vi "sub_log-header-write.vi"(7 "cmd":T1, 8 "error in (no error)":errorcluster, 11 "시험명":string) -> (0 "error out":errorcluster)   [LabVIEW 2019]
uses:
  log save type.ctl
  SubVIs/common/cmd_tablecnt.ctl
  _ctrl/rw.ctl
  _ctrl/create-rw-close.ctl
  Data Process/type-data.ctl
panel:
  out "Array":path[](array[path])
  out "dup path":path
  out "appended path":path
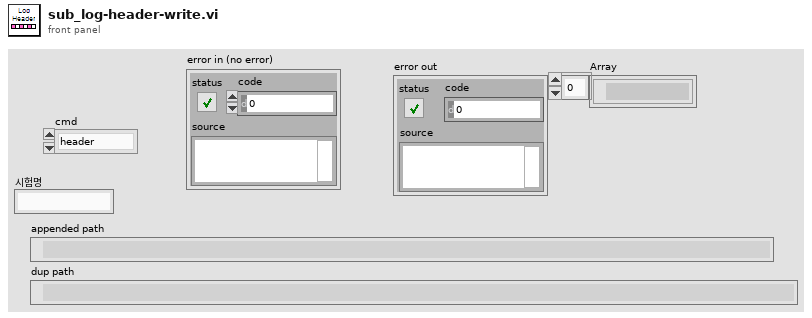
[diagram p1: front panel]
types:
  T1 = typedef "log save type.ctl" = enum16{"header", "data"}
  T2 = typedef "rw.ctl" = enum16{"read", "write"}
  T3 = typedef "cmd_tablecnt.ctl" = enum16{"Create", "Inital", "Write", "Default"}
  T4 = typedef "cap_config.ctl" = cluster{"Test Mode":enum32{"6.3.2 저온 작동/방치 시험", "6.3.3 고온 작동/방치 시험", "6.3.4 온도 싸이클 시험", "6.3.6 온습도 싸이클 시험", "6.3.8 결로 시험", "6.3.9 빙결 시험"}, "ON time[ms]":dbl, "OFF time[ms]":dbl, "1. 작동시간[분]":dbl, "2. 미작동시간[분]":dbl, "3. 작동시간[분]":dbl, "level[V]":dbl, "duty":dbl, "Freq":dbl, "Voltage+[V]":dbl, "Voltage-[V]":dbl, "Current+[A]":dbl, "Current-[A]":dbl, "출력전압[V]":dbl, "출력전류[A]":dbl, "OVP Level":dbl, "OCP Level":dbl, "Time Div":u16, "Record Len":i32, "방전 기준[V]":dbl, "Repeate (Each Ch)":u32, "Cycle[N]":u32, "ON/OFF 회 수[N]":dbl, "TrigPos[%]":dbl, "시험시간[분]":dbl}
  T5 = enum32{"6.3.2 저온 작동/방치 시험", "6.3.3 고온 작동/방치 시험", "6.3.4 온도 싸이클 시험", "6.3.6 온습도 싸이클 시험", "6.3.8 결로 시험", "6.3.9 빙결 시험"}
  T6 = typedef "Testing-info.ctl" = cluster{"전체채널수":u8, "현재채널번호":u8, "Irms":dbl, "입력전압":dbl, "입력전류":dbl, "출력전압":dbl, "출력전류":dbl, "온도":dbl, "제어단 단선":bool, "제어단 단락":bool, "제어단 특성변화":bool, "출력단 단선":bool, "출력단 단락":bool, "출력단 특성변화":bool, "출력단 전압":bool, "카운트 일치":bool, "Irms 판정":bool, "온도":bool, "테스트 회수":u32, "TestType":T7, "현재회수":u32, "Ch selection":cluster{"1ch":bool, "2ch":bool, "3ch":bool, "4ch":bool, "5ch":bool, "6ch":bool}, "반복":u32, "Path":path, "파일생성주기":u32, "start time":dbl, "stop time":dbl, "현재반복회수":u32, "NG":cluster{"입출력 카운트":bool, "출력전류RMS":bool}}
  T7 = typedef "sequence_single.ctl" = enum16{"Register", "RC", "B1", "B2", "B3", "Oper_LV", "Oper_HV", "ContR_LV"}
  T8 = typedef "type-data.ctl" = cluster{"dup path":path, "data":string}
  T9 = typedef "create-rw-close.ctl" = enum16{"create", "write", "read", "delete", "close"}
  T10 = cluster{"1ch":bool, "2ch":bool, "3ch":bool, "4ch":bool, "5ch":bool, "6ch":bool}
  T11 = typedef "result-path.ctl" = cluster{"Path-arr":path[]}
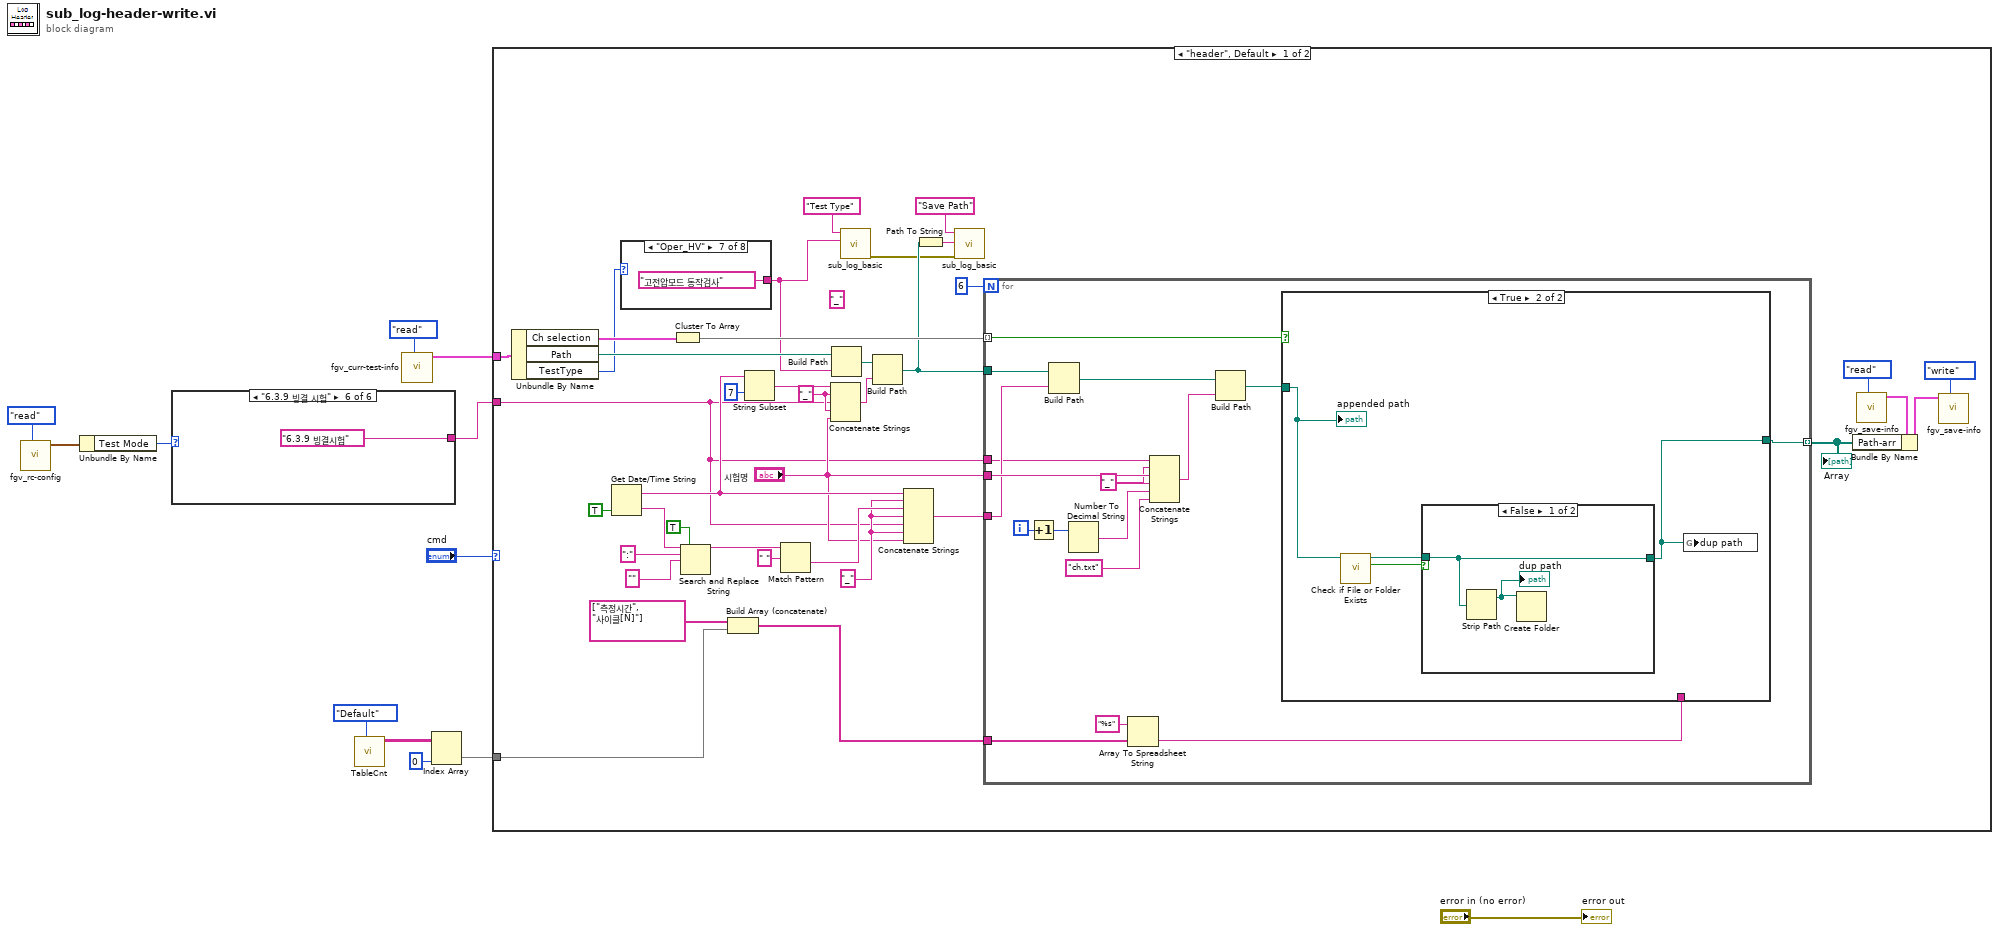
[diagram p0: block diagram]
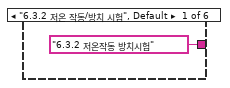
[diagram p2: hidden frame]
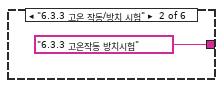
[diagram p3: hidden frame]
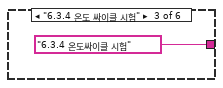
[diagram p4: hidden frame]
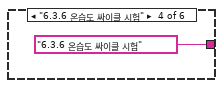
[diagram p5: hidden frame]
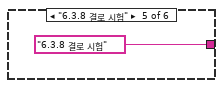
[diagram p6: hidden frame]
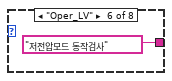
[diagram p12: hidden frame]
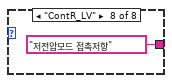
[diagram p13: hidden frame]
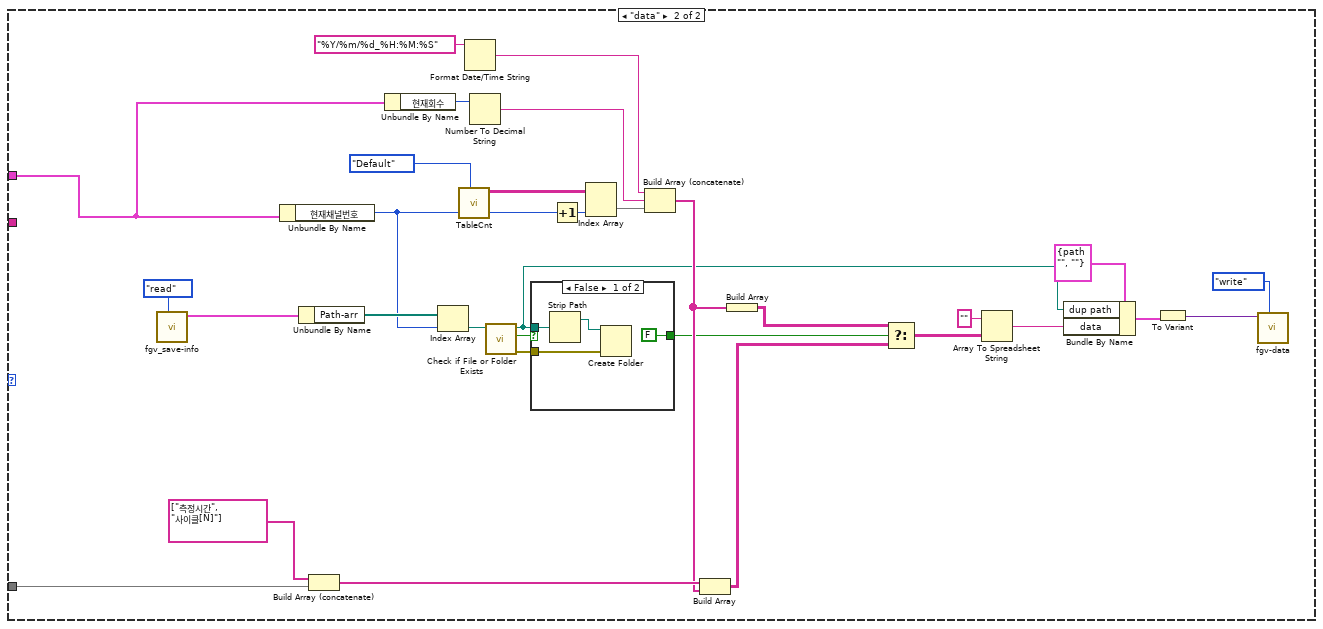
[diagram p16: hidden frame]
diagram:
  n1 = call "fgv_rc-config.vi"("cmd"=rw."read") -> ("Testconfig out"=w4:T4)  [unwired: 9 in, 1 out]
  n2 = Unbundle By Name(w4) -> ("Test Mode"=w2:T5)
  n3 = case shown="\"6.3.9 빙결 시험\"" w2 {
    tunnel: ["6.3.2 저온작동 방치시험" "6.3.3 고온작동 방치시험" "6.3.4 온도싸이클 시험" "6.3.6 온습도 싸이클 시험" "6.3.8 결로 시험" "6.3.9 빙결시험"] -> w1
    frame "6.3.2 저온 작동/방치 시험", Default {
    }
    frame "6.3.3 고온 작동/방치 시험" {
    }
    frame "6.3.4 온도 싸이클 시험" {
    }
    frame "6.3.6 온습도 싸이클 시험" {
    }
    frame "6.3.8 결로 시험" {
    }
    frame "6.3.9 빙결 시험" {
    }
  }
  n4 = call "TableCnt.vi"("cnt"=cmd_tablecnt."Default") -> ("Item Names"=w11:string[][])  [unwired: 9 in, 1 out]
  n5 = call "fgv_curr-test-info.vi"("cmd"=rw."read") -> ("현재테스트 정보 2"=w5:T6)  [unwired: 10 in]
  n6 = Index Array(array=w11, index (col)=0 ("disabled index (col)")) -> (element=w8:string[])  [unwired: 1 in]
  n7 = case shown="\"header\", Default" "cmd" {
    tunnel: w8 -> [w49 w104]
    tunnel: w5 -> [w27 w85]
    tunnel: w1 -> [w19 _]
    frame "header", Default {
      (unwired) "_" ("string")
      w24 = "_" ("string")
      w21 = "_" ("string")
      n8 = Unbundle By Name(w27) -> ("Ch selection"=w47:T10, "Path"=w38:path, "TestType"=w26:T7)
      n9 = Get Date/Time String(want seconds? (F)=TRUE) -> (date string=w23:string, time string=w45:string)  [unwired: 2 in]
      n10 = case shown="\"Oper_HV\"" w26 {
        tunnel: [_ _ _ _ _ "저전압모드 동작검사" ("Title") "고전압모드 동작검사" ("Title") "저전압모드 접촉저항" ("Title")] -> w25
        frame "Register", Default {
        }
        frame "RC" {
        }
        frame "B1" {
        }
        frame "B2" {
        }
        frame "B3" {
        }
        frame "Oper_LV" {
        }
        frame "Oper_HV" {
        }
        frame "ContR_LV" {
        }
      }
      n11 = Cluster To Array(cluster=w47) -> (array=w48:bool[])
      n12 = Search and Replace String(replace all?=TRUE ("replace all? (F)"), input string=w45, search string=":", replace string="" ("replace string (\"\")")) -> (result string=w41:string)  [unwired: 4 in, 3 out]
      n13 = Build Array (concatenate)(string[] ["측정시간", "사이클[N]"], w49) -> (w50:string[])
      n14 = String Subset(string=w23, length (rest)=7 ("length (rest)")) -> (substring=w30:string)  [unwired: 1 in]
      n15 = Match Pattern(string=w41, regular expression=" ") -> (after substring=w22:string)  [unwired: 1 in, 3 out]
      n16 = Concatenate Strings(w30, w24, w19, w24, "시험명") -> (w29:string)
      n17 = Build Path(base path=w38, name or relative path=w25) -> (appended path=w37:path)
      n18 = call "sub_log_basic.vi"("desc"=w25, "Title"="Test Type") -> ("error out"=w32:errorcluster)  [unwired: 9 in]
      n19 = Build Path(base path=w37, name or relative path=w29) -> (appended path=w34:path)
      n20 = Concatenate Strings(w23, w21, w22, w21, w19, w21, "시험명") -> (w28:string)
      n21 = Path To String(path=w34) -> (string=w35:string)
      n22 = call "sub_log_basic.vi"("error in"=w32, "desc"=w35, "Title"="Save Path") -> ()  [unwired: 8 in, 1 out]
      n23 = for {
        N: 6 -> [_]
        tunnel: w34 -> [w65]
        tunnel: [w67] -> w55 mode=indexing
        tunnel: w50 -> [w71]
        tunnel: w48 -> [w68] mode=indexing
        tunnel: "시험명" -> [w63]
        tunnel: w28 -> [w62]
        tunnel: w19 -> [w61]
        i -> [w76]
        w60 = "_" ("string")
        n24 = Increment(x=w76) -> (x+1=w69:i32)
        n25 = Build Path(base path=w65, name or relative path=w62) -> (appended path=w66:path)
        n26 = Number To Decimal String(number=w69) -> (decimal integer string=w75:string)  [unwired: 1 in]
        n27 = Array To Spreadsheet String(array=w71, 3:"%s" ("format string")) -> (spreadsheet string=w72:string)  [unwired: 1 in]
        n28 = Concatenate Strings(w61, w60, w63, w60, w75, "ch.txt" ("string")) -> (w64:string)
        n29 = Build Path(base path=w66, name or relative path=w64) -> (appended path=w73:path)
        n30 = case shown="True" w68 {
          tunnel: w73 -> [w77 w79]
          tunnel: w72 -> [_ _]
          tunnel: [w77 w78] -> w67
          frame False {
          }
          frame True {
            n31 = call <vilib>:"Check if File or Folder Exists.vi"("path"=w79) -> ("file or folder exists?"=w81:bool, "dup path"=w80:path)  [unwired: 8 in, 1 out]
            n32 = case shown="False" w81 {
              tunnel: w80 -> [w82 w84]
              tunnel: [w82 w84] -> w78
              frame False {
                n33 = Strip Path(path=w82) -> (stripped path=w83:path)  [unwired: 1 out]
                "dup path" <- w83
                n34 = Create Folder(path (use dialog)=w83) -> ()  [unwired: 2 in, 3 out]
              }
              frame True {
              }
            }
            n35 = global write "Global_내구.vi" "dup path"(w78) -> ()
            "appended path" <- w79
          }
        }
      }
      "Array" <- w55
      n36 = call "fgv_save-info.vi"("cmd"=rw."read") -> ("save info 2"=w54:T11)  [unwired: 10 in]
      n37 = Bundle By Name(cluster=w54, "Path-arr"=w55) -> (w56:T11)
      n38 = call "fgv_save-info.vi"("cmd"=rw."write", "save info"=w56) -> ()  [unwired: 9 in, 1 out]
    }
    frame "data" {
      n39 = call "fgv_save-info.vi"("cmd"=rw."read") -> ("save info 2"=w114:T11)  [unwired: 10 in]
      n40 = Unbundle By Name(w85) -> ("현재채널번호"=w109:u8)
      n41 = Unbundle By Name(w114) -> ("Path-arr"=w113:path[])
      n42 = Build Array (concatenate)(string[] ["측정시간", "사이클[N]"], w104) -> (w103:string[])
      n43 = Unbundle By Name(w85) -> ("현재회수"=w107:u32)
      n44 = Index Array(array=w113, index=w109) -> (element=w105:path)
      n45 = call "TableCnt.vi"("cnt"=cmd_tablecnt."Default") -> ("Item Names"=w110:string[][])  [unwired: 9 in, 1 out]
      n46 = Format Date/Time String(time format string (%c)="%Y/%m/%d_%H:%M:%S") -> (date/time string=w86:string)  [unwired: 2 in]
      n47 = Number To Decimal String(number=w107) -> (decimal integer string=w87:string)  [unwired: 1 in]
      n48 = call <vilib>:"Check if File or Folder Exists.vi"("path"=w105) -> ("error out"=w98:errorcluster, "file or folder exists?"=w99:bool, "dup path"=w93:path)  [unwired: 8 in]
      n49 = case shown="False" w99 {
        selector: w99 -> [_ w120]
        tunnel: w93 -> [w118 _]
        tunnel: w98 -> [w117 _]
        tunnel: [FALSE w120] -> w97
        frame False {
          n50 = Strip Path(path=w118) -> (stripped path=w119:path)  [unwired: 1 out]
          n51 = Create Folder(path (use dialog)=w119, error in=w117) -> ()  [unwired: 1 in, 3 out]
        }
        frame True {
        }
      }
      n52 = Increment(x=w109) -> (x+1=w108:u8)
      n53 = Index Array(array=w110, index (col)=w108) -> (element=w106:string[])  [unwired: 1 in]
      n54 = Build Array (concatenate)(w86, w87, w106) -> (w102:string[])
      n55 = Build Array(w103, w102) -> (w95:string[][])
      n56 = Build Array(w102) -> (w96:string[][])
      n57 = Select(t=w96, s=w97, f=w95) -> (s? t:f=w101:string[][])
      n58 = Array To Spreadsheet String(array=w101, 3:"" ("format string")) -> (spreadsheet string=w92:string)  [unwired: 1 in]
      n59 = Bundle By Name(cluster=T8 {"dup path"=path "", "data"=""}, "dup path"=w93, "data"=w92) -> (w91:T8)
      n60 = To Variant(anything=w91) -> (Variant=w90:variant)
      n61 = call "fgv-data.vi"("cmd"=create-rw-close."write", "element"=w90) -> ()  [unwired: 8 in, 2 out]
    }
  }
  "error out" <- "error in (no error)"
